vi "Initialize Stimulator.vi"(4 "error in (no error)":errorcluster, 7 "Stimulator":T1={"Stim Open Data"={"Name"="", "Mode"=enum."LIVE", "Visa Timeout"=0}, "Stim Init Data"={"Frequency"=0.0, "N Factor"=0, "D/T Int"=0.0, "Active Channels"=[], "LF Channels"=[]}, "Stim Update Data"={"Pulse Mode"=[enum."Single"], "Current"=[], "Pulse Dur"=[]}, "Stim Status"={"Open"=FALSE, "On"=FALSE}}) -> (0 "error out":errorcluster, 1 "Write to Log":string, 2 "Response":u8, 3 "Stimulator":T1={"Stim Open Data"={"Name"="", "Mode"=enum."LIVE", "Visa Timeout"=0}, "Stim Init Data"={"Frequency"=0.0, "N Factor"=0, "D/T Int"=0.0, "Active Channels"=[FALSE], "LF Channels"=[]}, "Stim Update Data"={"Pulse Mode"=[], "Current"=[], "Pulse Dur"=[]}, "Stim Status"={"Open"=FALSE, "On"=FALSE}})   [LabVIEW 2019]
doc: "Use this template to build a VI to use as a subVI."
uses:
  Data Type Defs/Stimulator.ctl
  Data Type Defs/Stim Open Data.ctl
  Data Type Defs/Stim Init Data.ctl
  Data Type Defs/Stim Update Data.ctl
  Data Type Defs/Pulse Mode (array).ctl
  Data Type Defs/Stim Status.ctl
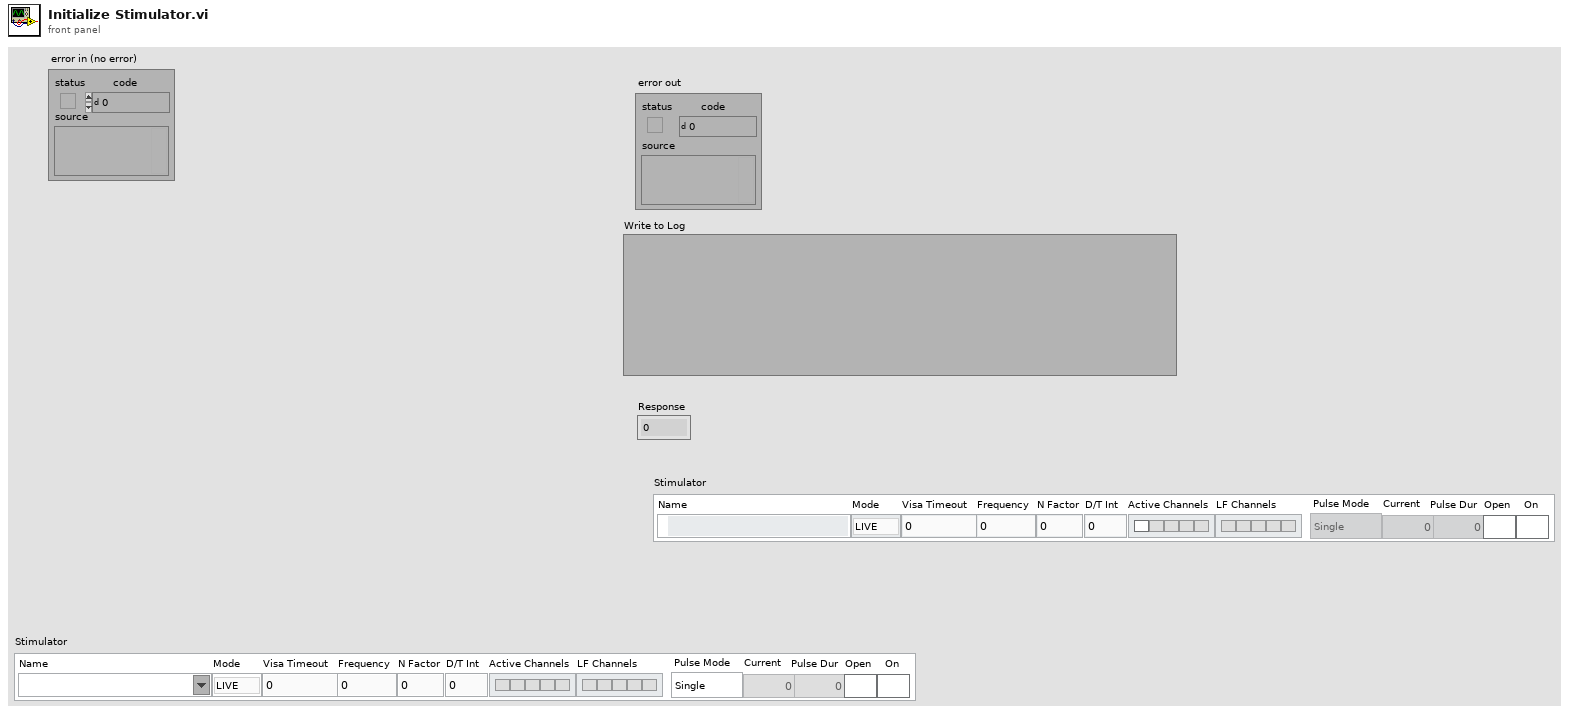
[diagram p1: front panel]
types:
  T1 = typedef "Stimulator.ctl" = cluster{"Stim Open Data":T2, "Stim Init Data":T3, "Stim Update Data":T4, "Stim Status":T6}
  T2 = typedef "Stim Open Data.ctl" = cluster{"Name":refnum<visa-resource-name>, "Mode":enum16{"LIVE", "SIM"}, "Visa Timeout":u32}
  T3 = typedef "Stim Init Data.ctl" = cluster{"Frequency":dbl, "N Factor":u8, "D/T Int":dbl, "Active Channels":bool[], "LF Channels":bool[]}
  T4 = typedef "Stim Update Data.ctl" = cluster{"Pulse Mode":T5, "Current":u32[], "Pulse Dur":u32[]}
  T5 = typedef "Pulse Mode (array).ctl" = enum16{"Single", "Doublet", "Triplet"}[]
  T6 = typedef "Stim Status.ctl" = cluster{"Open":bool, "On":bool}
  T7 = cluster{"Command Name":string, "Command String":string, "Log String":string}
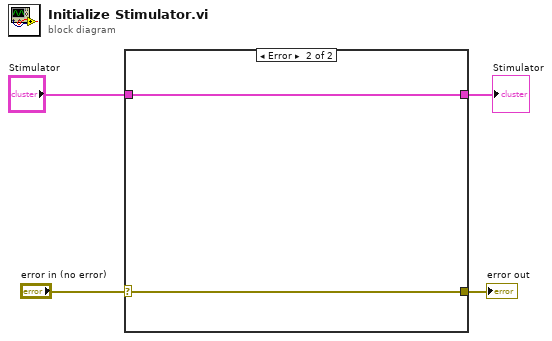
[diagram p0: block diagram]
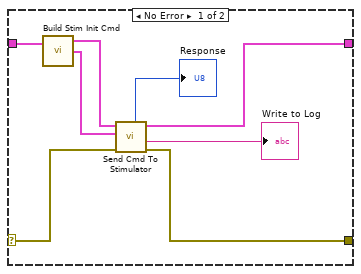
[diagram p2: hidden frame]
diagram:
  n1 = case shown="Error" "error in (no error)" {
    selector: "error in (no error)" -> [w10 w14]
    tunnel: [w9 w14] -> w3
    tunnel: "Stimulator" -> [w5 w13]
    tunnel: [w6 w13] -> w2
    frame No Error {
      n2 = call "Build Stim Init Cmd.vi"("Stimulator"=w5) -> ("Stimulator"=w8:T1, "Command"=w7:T7)  [unwired: 2 in]
      n3 = call "Send Cmd To Stimulator.vi"("Stimulator"=w8, "Command"=w7, "error in (no error)"=w10) -> ("Numeric Response"=→"Response":u8, "Stimulator"=w6:T1, "Log Entry"=→"Write to Log":string, "error out"=w9:errorcluster)  [unwired: 1 in, 1 out]
    }
    frame Error {
    }
  }
  "error out" <- w3
  "Stimulator" <- w2
